vi "stim line entry cluster refnum split (sub-vi).vi"(8 "error in (no error)":errorcluster, 11 "stim. config line cluster refnum":refnum<vi>) -> (0 "error out":errorcluster, 2 "element refnum cluster":T1, 3 "stim. config line cluster refnum out":refnum<vi>)   [LabVIEW 2021]
uses:
  type-defs/stimulator configuration line cluster (type def).ctl
  type-defs/port-odor with color cluster (type def).ctl
  type-defs/port-odor ring (type def).ctl
  type-defs/odor color (type def).ctl
panel:
  in  "stim. config line":T2={"description"="", "duration, s"=0.0, "left odor"={"port-odor ring"=0, "odor color"=9}, "middle odor"={"port-odor ring"=0, "odor color"=9}, "right odor"={"port-odor ring"=0, "odor color"=9}, "selected?"=FALSE} {"right odor"."port-odor ring" items=["off"]; "middle odor"."port-odor ring" items=["off"]; "left odor"."port-odor ring" items=["off"]}
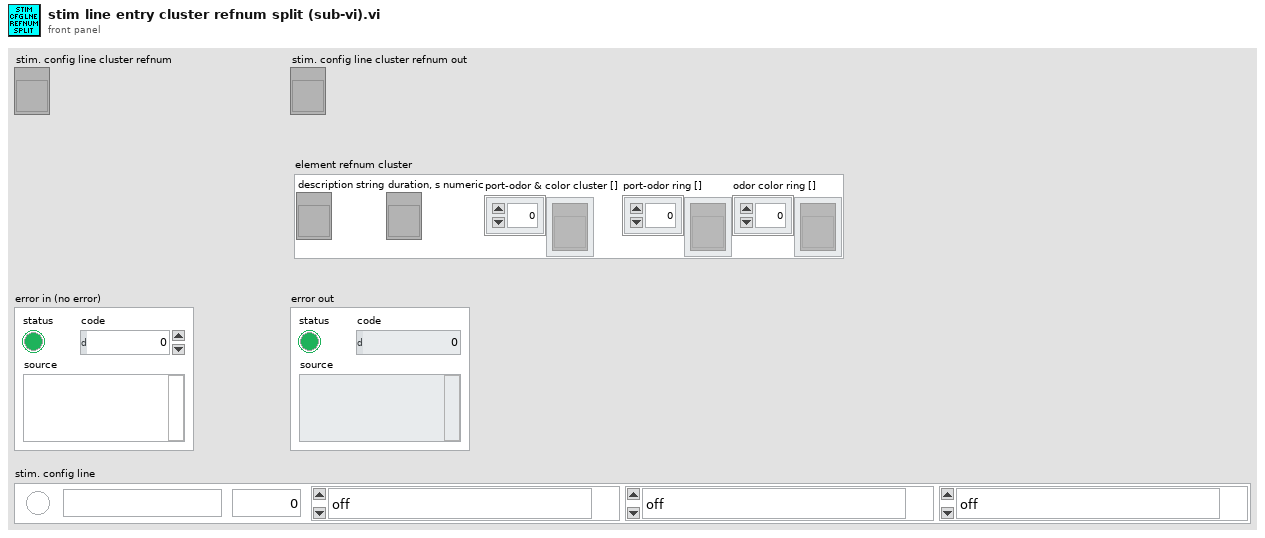
[diagram p1: front panel]
types:
  T1 = cluster{"description string":refnum<vi>, "duration, s numeric":refnum<vi>, "port-odor & color cluster []":refnum<vi>[], "port-odor ring []":refnum<vi>[], "odor color ring []":refnum<vi>[]}
  T2 = typedef "stimulator configuration line cluster (type def).ctl" = cluster{"description":string, "duration, s":dbl, "left odor":T3, "middle odor":T3, "right odor":T3, "selected?":bool}
  T3 = typedef "port-odor with color cluster (type def).ctl" = cluster{"port-odor ring":T4, "odor color":T5}
  T4 = typedef "port-odor ring (type def).ctl" = u16
  T5 = typedef "odor color (type def).ctl" = u16
  T6 = cluster{"port-odor ring":refnum<vi>, "odor color ring":refnum<vi>}
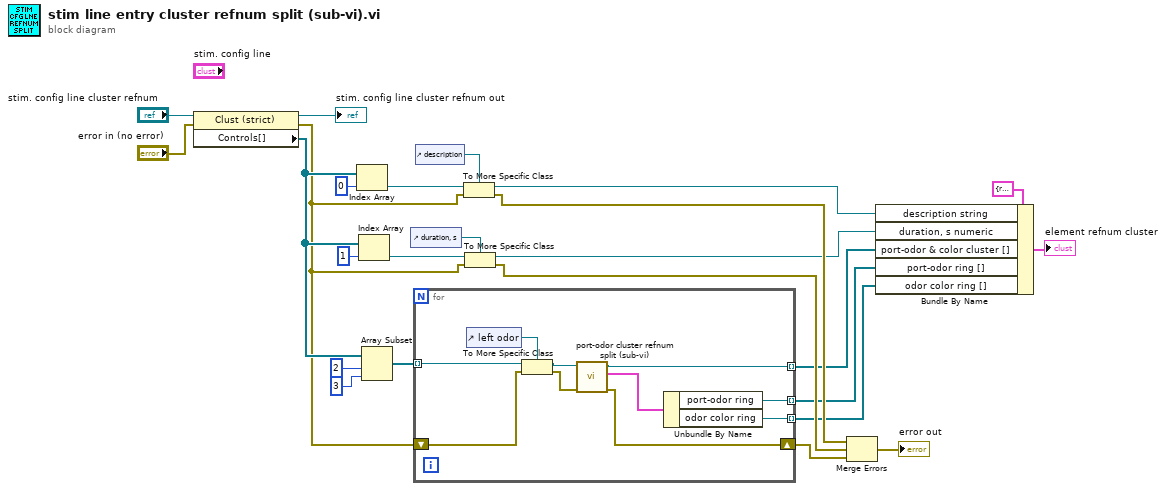
[diagram p0: block diagram]
diagram:
  n1 = property class="Clust (strict)"(reference="stim. config line cluster refnum", error in="error in (no error)") -> (reference out=→"stim. config line cluster refnum out":refnum<vi>, error out=w15:errorcluster, "Controls[]"=w22:refnum<vi>[])
  n2 = Index Array(array=w22, index=0) -> (element=w20:refnum<vi>)
  n3 = Index Array(array=w22, index=1) -> (element=w17:refnum<vi>)
  n4 = Array Subset(array=w22, index=2, length=3) -> (w16:refnum<vi>[])
  n5 = control-ref of="duration, s"() -> (w18:refnum<vi>)
  n6 = for {
    tunnel: w16 -> [w34] mode=indexing
    tunnel: [w32] -> w7 mode=indexing
    shift-right: [w30] -> w14
    shift-left: w15 -> [w29]
    tunnel: [w27] -> w6 mode=indexing
    tunnel: [w26] -> w5 mode=indexing
    n7 = control-ref of="left odor"() -> (w35:refnum<vi>)
    n8 = To More Specific Class(target class=w35, reference=w34, error in=w29) -> (specific class reference=w33:refnum<vi>, error out=w31:errorcluster)
    n9 = call "port-odor cluster refnum split (sub-vi).vi"("error in (no error)"=w31, "port-odor and color cluster refnum"=w33) -> ("error out"=w30:errorcluster, "element refnum cluster"=w28:T6, "port-odor and color cluster refnum out"=w32:refnum<vi>)  [unwired: 7 in]
    n10 = Unbundle By Name(w28) -> ("port-odor ring"=w27:refnum<vi>, "odor color ring"=w26:refnum<vi>)
  }
  n11 = control-ref of="description"() -> (w19:refnum<vi>)
  n12 = To More Specific Class(target class=w19, reference=w20, error in=w15) -> (specific class reference=w9:refnum<vi>, error out=w11:errorcluster)
  n13 = To More Specific Class(target class=w18, reference=w17, error in=w15) -> (specific class reference=w8:refnum<vi>, error out=w12:errorcluster)
  n14 = Merge Errors(w11, w12, w14) -> (→"error out":errorcluster)
  n15 = Bundle By Name(cluster=T1 {"description string"=refnum, "duration, s numeric"=refnum, "port-odor & color cluster []"=[], "port-odor ring []"=[], "odor color ring []"=[]} ("element refnum cluster"), "description string"=w9, "duration, s numeric"=w8, "port-odor & color cluster []"=w7, "port-odor ring []"=w6, "odor color ring []"=w5) -> (→"element refnum cluster":T1)
